vi "slide controller.vi"(7 "slide action":T1, 11 "slide control":refnum<vi>) -> (0 "in slide":bool, 1 "slide control OUT":T2, 3 "slide control OUT":refnum<vi>, 4 "halt event":bool)   [LabVIEW 2015]
uses:
  slide control.ctl
  slide action.ctl
  follow the peak action.ctl
panel:
  in  "slide control":T2
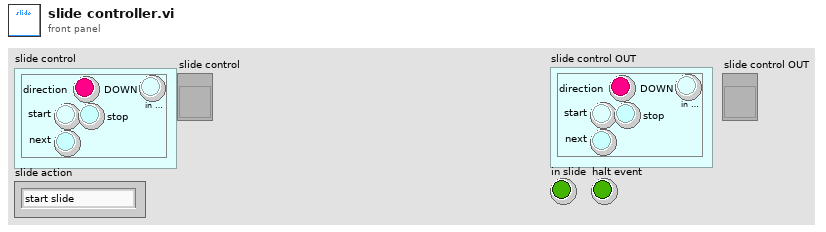
[diagram p1: front panel]
types:
  T1 = typedef "slide action.ctl" = enum16{"start slide", "stop slide", "init", "check", "halt", "un-next", "next", "run", "slide UP", "slide DOWN"}
  T2 = typedef "slide control.ctl" = cluster{"in slide":bool, "direction":bool, "start ":bool, "stop":bool, "next":bool}
  T3 = typedef "follow the peak action.ctl" = enum16{"make clean", "make dirty", "follow the peak", "unfollow the peak", "follow gamma", "unfollow gamma", "check", "toggle omega", "toggle gamma"}
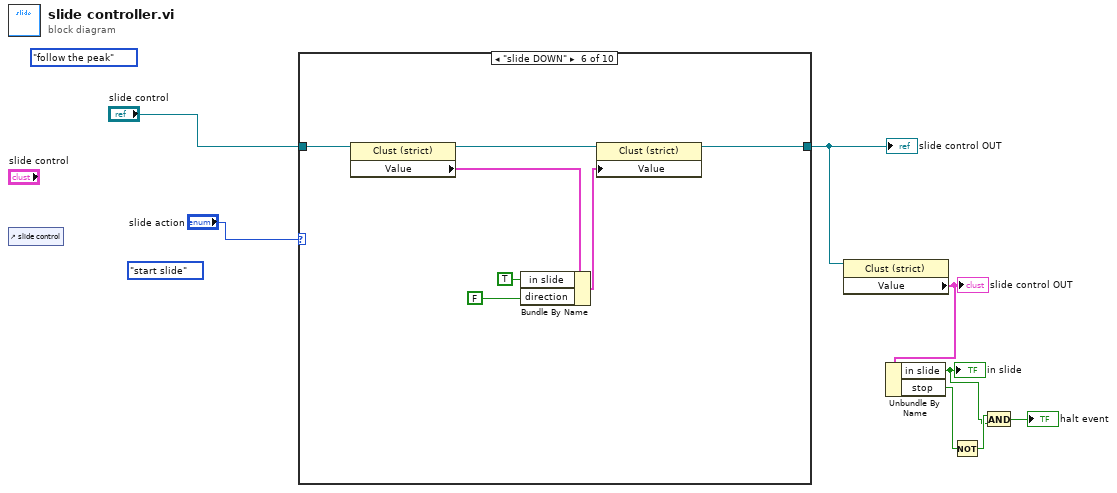
[diagram p0: block diagram]
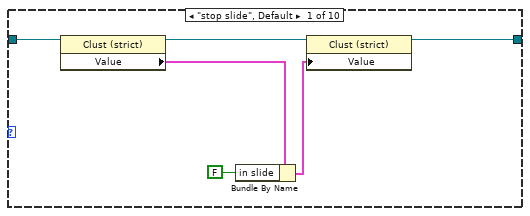
[diagram p2: hidden frame]
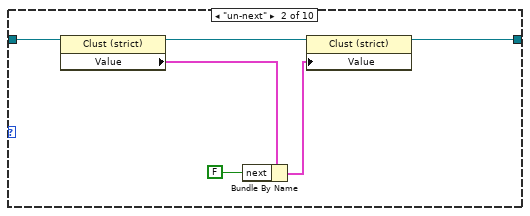
[diagram p3: hidden frame]
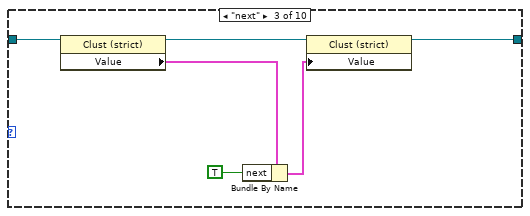
[diagram p4: hidden frame]
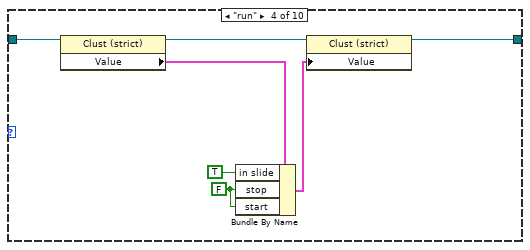
[diagram p5: hidden frame]
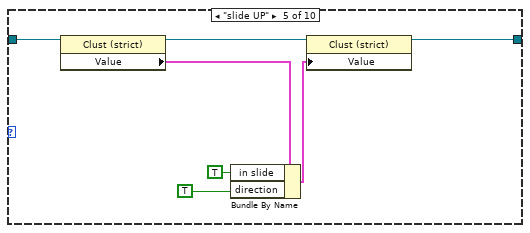
[diagram p6: hidden frame]
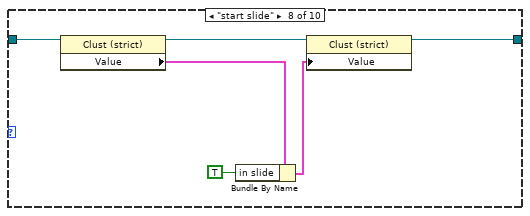
[diagram p8: hidden frame]
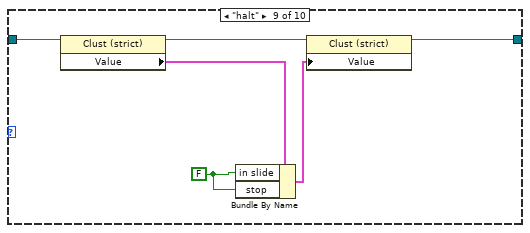
[diagram p9: hidden frame]
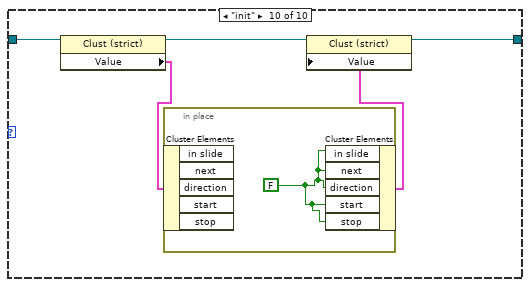
[diagram p10: hidden frame]
diagram:
  (unwired) slide_action."start slide" ("action")
  (unwired) follow_the_peak_action."follow the peak" ("action")
  n1 = control-ref of="slide control"() -> ()  [unwired: 1 out]
  n2 = case shown="\"slide DOWN\"" "slide action" {
    tunnel: "slide control" -> [w14 w20 w26 w33 w40 w47 w48 w54 w60 w65]
    tunnel: [w11 w17 w23 w30 w37 w44 w48 w51 w57 w63] -> w8
    frame "stop slide", Default {
      n3 = property class="Clust (strict)"(reference=w14) -> (reference out=w12:refnum<vi>, "Value"=w13:T2)  [unwired: 1 in, 1 out]
      n4 = Bundle By Name(cluster=w13, "in slide"=FALSE ("omega ?")) -> (w10:T2)
      n5 = property class="Clust (strict)"(reference=w12, "Value"=w10) -> (reference out=w11:refnum<vi>)  [unwired: 1 in, 1 out]
    }
    frame "un-next" {
      n6 = property class="Clust (strict)"(reference=w20) -> (reference out=w18:refnum<vi>, "Value"=w19:T2)  [unwired: 1 in, 1 out]
      n7 = Bundle By Name(cluster=w19, "next"=FALSE ("omega ?")) -> (w16:T2)
      n8 = property class="Clust (strict)"(reference=w18, "Value"=w16) -> (reference out=w17:refnum<vi>)  [unwired: 1 in, 1 out]
    }
    frame "next" {
      n9 = property class="Clust (strict)"(reference=w26) -> (reference out=w24:refnum<vi>, "Value"=w25:T2)  [unwired: 1 in, 1 out]
      n10 = Bundle By Name(cluster=w25, "next"=TRUE ("omega ?")) -> (w22:T2)
      n11 = property class="Clust (strict)"(reference=w24, "Value"=w22) -> (reference out=w23:refnum<vi>)  [unwired: 1 in, 1 out]
    }
    frame "run" {
      w27 = FALSE ("stop")
      n12 = property class="Clust (strict)"(reference=w33) -> (reference out=w31:refnum<vi>, "Value"=w32:T2)  [unwired: 1 in, 1 out]
      n13 = Bundle By Name(cluster=w32, "in slide"=TRUE ("omega ?"), "stop"=w27, "start"=w27) -> (w29:T2)
      n14 = property class="Clust (strict)"(reference=w31, "Value"=w29) -> (reference out=w30:refnum<vi>)  [unwired: 1 in, 1 out]
    }
    frame "slide UP" {
      n15 = property class="Clust (strict)"(reference=w40) -> (reference out=w38:refnum<vi>, "Value"=w39:T2)  [unwired: 1 in, 1 out]
      n16 = Bundle By Name(cluster=w39, "in slide"=TRUE ("omega ?"), "direction"=TRUE ("stop")) -> (w36:T2)
      n17 = property class="Clust (strict)"(reference=w38, "Value"=w36) -> (reference out=w37:refnum<vi>)  [unwired: 1 in, 1 out]
    }
    frame "slide DOWN" {
      n18 = property class="Clust (strict)"(reference=w47) -> (reference out=w45:refnum<vi>, "Value"=w46:T2)  [unwired: 1 in, 1 out]
      n19 = Bundle By Name(cluster=w46, "in slide"=TRUE ("omega ?"), "direction"=FALSE ("stop")) -> (w43:T2)
      n20 = property class="Clust (strict)"(reference=w45, "Value"=w43) -> (reference out=w44:refnum<vi>)  [unwired: 1 in, 1 out]
    }
    frame "check" {
    }
    frame "start slide" {
      n21 = property class="Clust (strict)"(reference=w54) -> (reference out=w52:refnum<vi>, "Value"=w53:T2)  [unwired: 1 in, 1 out]
      n22 = Bundle By Name(cluster=w53, "in slide"=TRUE ("omega ?")) -> (w50:T2)
      n23 = property class="Clust (strict)"(reference=w52, "Value"=w50) -> (reference out=w51:refnum<vi>)  [unwired: 1 in, 1 out]
    }
    frame "halt" {
      w55 = FALSE ("omega ?")
      n24 = property class="Clust (strict)"(reference=w60) -> (reference out=w58:refnum<vi>, "Value"=w59:T2)  [unwired: 1 in, 1 out]
      n25 = Bundle By Name(cluster=w59, "in slide"=w55, "stop"=w55) -> (w56:T2)
      n26 = property class="Clust (strict)"(reference=w58, "Value"=w56) -> (reference out=w57:refnum<vi>)  [unwired: 1 in, 1 out]
    }
    frame "init" {
      n27 = property class="Clust (strict)"(reference=w65) -> (reference out=w64:refnum<vi>, "Value"=w62:T2)  [unwired: 1 in, 1 out]
      n28 = in-place {
        w66 = FALSE ("Boolean")
        n29 = in-place-cluster #1(w62) -> ()  [unwired: 5 out]
        n30 = in-place-cluster #1("in slide"=w66, "next"=w66, "direction"=w66, "start"=w66, "stop"=w66) -> (w61:T2)
      }
      n31 = property class="Clust (strict)"(reference=w64, "Value"=w61) -> (reference out=w63:refnum<vi>)  [unwired: 1 in, 1 out]
    }
  }
  "slide control OUT" <- w8
  n32 = property class="Clust (strict)"(reference=w8) -> ("Value"=w5:T2)  [unwired: 1 in, 2 out]
  "slide control OUT" <- w5
  n33 = Unbundle By Name(w5) -> ("in slide"=w2:bool, "stop"=w3:bool)
  "in slide" <- w2
  n34 = Not(x=w3) -> (.not. x?=w4:bool)
  n35 = And(x=w4, y=w2) -> (x .and. y?=→"halt event":bool)
